vi "Utility - Display One Button Dialog if NOT Blank.vi"(9 "Button Name (OK)":string="OK", 10 "message":string) -> (2 "Msg Done":bool)   [LabVIEW 2014]
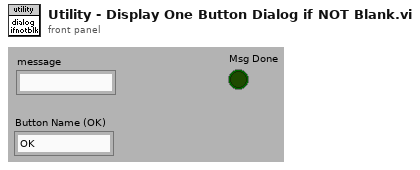
[diagram p1: front panel]
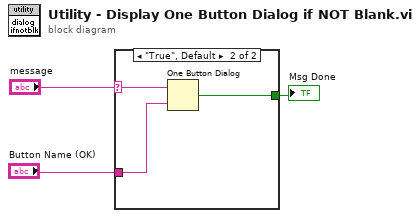
[diagram p0: block diagram]
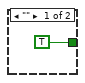
[diagram p2: hidden frame]
diagram:
  n1 = case shown="\"True\", Default" "message" {
    selector: "message" -> [_ w5]
    tunnel: "Button Name (OK)" -> [_ w7]
    tunnel: [TRUE ("true") w6] -> w2
    frame "" {
    }
    frame "True", Default {
      n2 = One Button Dialog(message=w5, button name ("OK")=w7) -> (true=w6:bool)
    }
  }
  "Msg Done" <- w2
